vi "Untitled 1.vi"() -> ()   [LabVIEW 2016]
panel:
  out "Boolean":bool
  out "output variable":dbl format="%_9f"
  in  "X":dbl
  in  "m":dbl
  in  "Для запуска программы установите 1":dbl
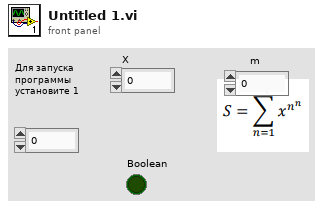
[diagram p1: front panel]
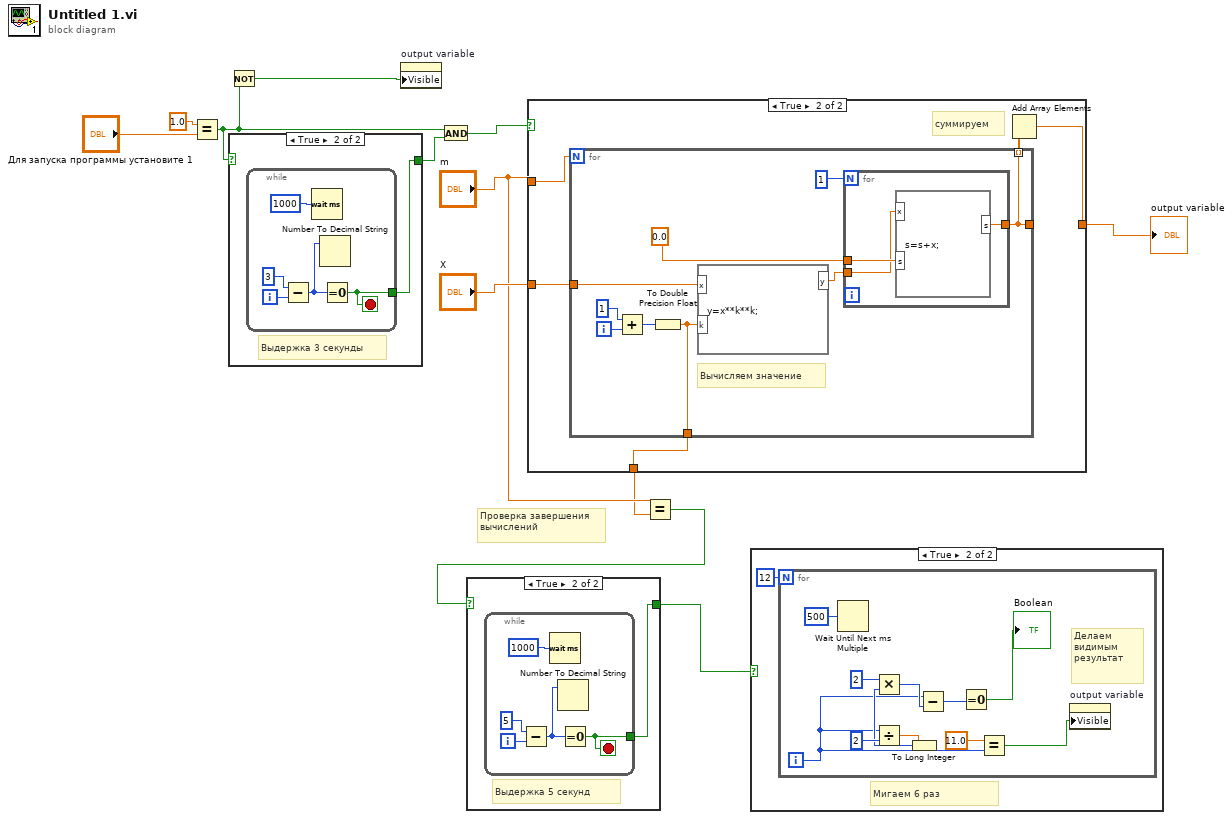
[diagram p0: block diagram]
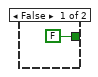
[diagram p2: hidden frame]
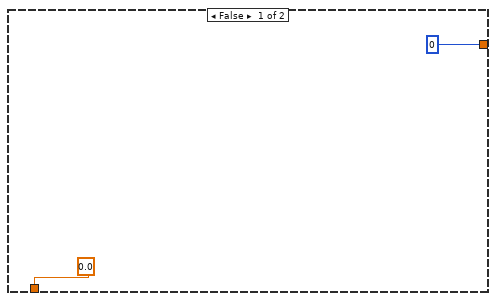
[diagram p4: hidden frame]
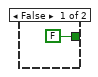
[diagram p5: hidden frame]
diagram:
  # "Проверка завершения вычислений"
  n1 = Equal?(x=1.0, y="Для запуска программы установите 1") -> (x = y?=w2:bool)
  n2 = Not(x=w2) -> (.not. x?=w1:bool)
  n3 = case shown="True" w2 {
    tunnel: [FALSE w14] -> w9
    frame False {
    }
    frame True {
      # "Выдержка 3 секунды"
      n4 = while {
        tunnel: [w15] -> w14
        i -> [w18]
        stop <- w15 stop-if-true
        n5 = Subtract(x=3, y=w18) -> (x-y=w16:i32)
        n6 = Wait (ms)(milliseconds to wait=u32 1000) -> ()  [unwired: 1 out]
        n7 = Number To Decimal String(number=w16) -> ()  [unwired: 1 in, 1 out]
        n8 = Equal To 0?(x=w16) -> (x = 0?=w15:bool)
      }
    }
  }
  n9 = property on="output variable" class="DigNum (strict)"("Visible"=w1) -> ()  [unwired: 2 in, 2 out]
  n10 = And(x=w2, y=w9) -> (x .and. y?=w8:bool)
  n11 = case shown="True" w8 {
    tunnel: "m" -> [_ w25]
    tunnel: "X" -> [_ w26]
    tunnel: [0 w23] -> w7
    tunnel: [0.0 w22] -> w5
    frame False {
    }
    frame True {
      # "суммируем"
      n12 = for {
        N: w25 -> [_]
        tunnel: w26 -> [w35]
        tunnel: [w28] -> _
        tunnel: [w28] -> w24 mode=indexing
        tunnel: [w27] -> w22
        i -> [w34]
        # "Вычисляем значение"
        n13 = Add(x=1, y=w34) -> (x+y=w32:i32)
        n14 = To Double Precision Float(number=w32) -> (double precision float=w27:dbl)
        n15 = formula code="y=x**k**k;"("x"=w35, "k"=w27) -> ("y"=w30:dbl)
        n16 = for {
          N: 1 -> [_]
          tunnel: [w38] -> w28
          tunnel: w30 -> [w36]
          tunnel: 0.0 -> [w37]
          n17 = formula code="s=s+x;"("x"=w36, "s"=w37) -> ("s"=w38:dbl)
        }
      }
      n18 = Add Array Elements(numeric array=w24) -> (sum=w23:dbl)
    }
  }
  "output variable" <- w7
  n19 = Equal?(x="m", y=w5) -> (x = y?=w4:bool)
  n20 = case shown="True" w4 {
    tunnel: [FALSE w40] -> w3
    frame False {
    }
    frame True {
      # "Выдержка 5 секунд"
      n21 = while {
        tunnel: [w41] -> w40
        i -> [w44]
        stop <- w41 stop-if-true
        n22 = Subtract(x=5, y=w44) -> (x-y=w42:i32)
        n23 = Wait (ms)(milliseconds to wait=u32 1000) -> ()  [unwired: 1 out]
        n24 = Number To Decimal String(number=w42) -> ()  [unwired: 1 in, 1 out]
        n25 = Equal To 0?(x=w42) -> (x = 0?=w41:bool)
      }
    }
  }
  n26 = case shown="True" w3 {
    frame False {
    }
    frame True {
      # "Мигаем 6 раз"
      n27 = for {
        N: 12 -> [_]
        i -> [w48]
        # "Делаем видимым результат"
        n28 = Wait Until Next ms Multiple(millisecond multiple=u32 500) -> ()  [unwired: 1 out]
        n29 = Divide(x=w48, y=2) -> (x/y=w56:dbl)
        n30 = To Long Integer(number=w56) -> (32bit integer=w55:i32)
        n31 = Multiply(x=2, y=w55) -> (x*y=w53:i32)
        n32 = Subtract(x=w48, y=w53) -> (x-y=w52:i32)
        n33 = Equal To 0?(x=w52) -> (x = 0?=→"Boolean":bool)
        n34 = Equal?(x=11.0, y=w48) -> (x = y?=w47:bool)
        n35 = property on="output variable" class="DigNum (strict)"("Visible"=w47) -> ()  [unwired: 2 in, 2 out]
      }
    }
  }
